vi "DQMH Request UI Display.vi"(7 "Module DIsk Path":path, 8 "error in (no error)":errorcluster, 9 "Display Scenario":T1, 11 "Application reference":refnum<vi>) -> (0 "error out":errorcluster, 3 "Accept?":bool)   [LabVIEW 2020, in "hse-dqmh-dynamicrequesters.lvlib"]
doc: "Calls the \"Request UI Display\" request VI of the module in <b>Path to module directory</b>. Hands over the <b>Module Name</b> and the <b>Display Scenario</b>.\n\n____\nHAMPEL SOFTWARE ENGINEERING v3.8.0 (2023-12-18 14:41)"
uses:
  hse-dqmh-dynamicrequesters.lvlib
  Controls/Module Display Scenarios.ctl
  hse-dqmh.lvlib
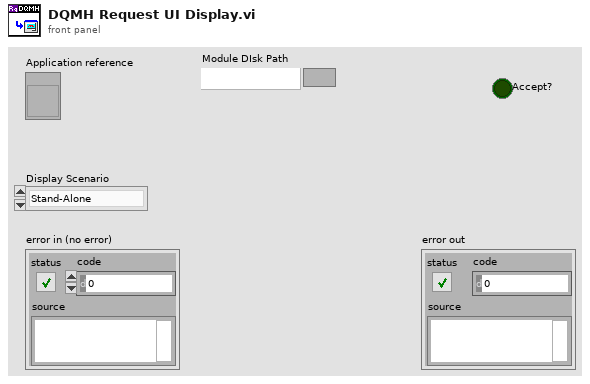
[diagram p1: front panel]
types:
  T1 = typedef "hse-dqmh.lvlib/Module Display Scenarios.ctl" = enum16{"Stand-Alone", "Managed"}
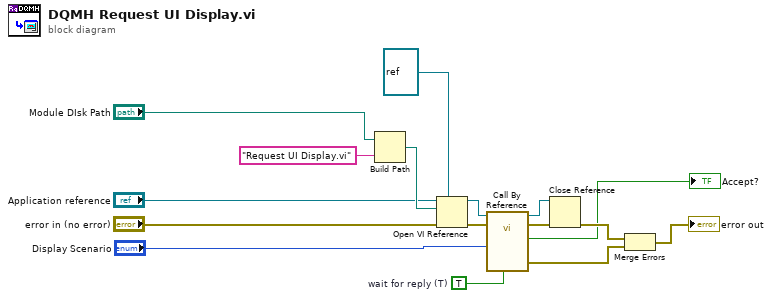
[diagram p0: block diagram]
diagram:
  w2 = TRUE  # wait for reply (T)
  n1 = Build Path(base path="Module DIsk Path", name or relative path="Request UI Display.vi") -> (appended path=w14:path)
  n2 = Open VI Reference(type specifier VI Refnum (for type only)=refnum<vi> refnum, application reference (local)="Application reference", vi path=w14, error in (no error)="error in (no error)") -> (vi reference=w16:refnum<vi>, error out=w11:errorcluster)  [unwired: 2 in]
  n3 = call-by-ref "?"(reference=w16, error in=w11, "wait for reply (T)"=w2, "Scenario"="Display Scenario") -> (reference out=w8:refnum<vi>, error out=w12:errorcluster, 0:"error out"=w13:errorcluster, "Accept?"=→"Accept?":bool)  [unwired: 8 in]
  n4 = Close Reference(reference=w8, error in (no error)=w12) -> (error out=w9:errorcluster)
  n5 = Merge Errors(w9, w13) -> (→"error out":errorcluster)
